vi "Generate File Header.vi"() -> ()   [LabVIEW 2012]
uses:
  Header Data.ctl
panel:
  out "File Header":string
  in  "File Header Data":T1={"Operator Name"="Fred", "UUT Serial Number"="A001", "Test Name"="Test System"}
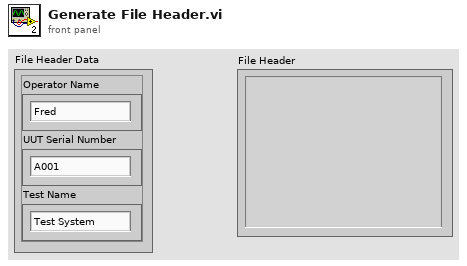
[diagram p1: front panel]
types:
  T1 = typedef "Header Data.ctl" = cluster{"Operator Name":string, "UUT Serial Number":string, "Test Name":string}
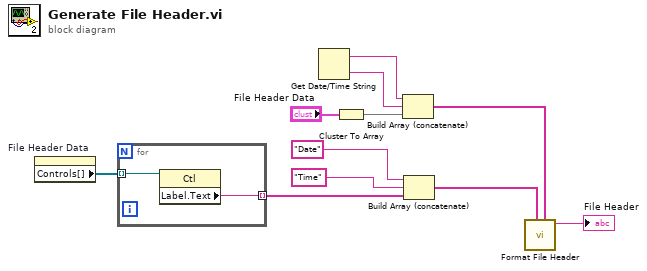
[diagram p0: block diagram]
diagram:
  n1 = property on="File Header Data" class="Clust (strict)"() -> ("Controls[]"=w10:refnum<vi>[])  [unwired: 2 in, 2 out]
  n2 = for {
    tunnel: w10 -> [w13] mode=indexing
    tunnel: [w12] -> w8 mode=indexing
    n3 = property class="Ctl"(reference=w13) -> ("Label.Text"=w12:string)  [unwired: 1 in, 2 out]
  }
  n4 = Get Date/Time String() -> (date string=w4:string, time string=w5:string)  [unwired: 3 in]
  n5 = Cluster To Array(cluster="File Header Data") -> (array=w9:string[])
  n6 = Build Array (concatenate)(w4, w5, w9) -> (w2:string[])
  n7 = Build Array (concatenate)("Date", "Time", w8) -> (w3:string[])
  n8 = call "Format File Header.vi"("Header Data (Empty)"=w2, "Header Titles (Empty)"=w3) -> ("File Header"=→"File Header":string)  [unwired: 8 in, 1 out]
